vi "ObtainBroadcastEvents.vi"(8 "error in (no error)":errorcluster) -> (0 "error out":errorcluster, 2 "clBroadcastEvents":T1)   [LabVIEW 2017, in "EventModule.lvlib"]
uses:
  EventModule.lvlib
  clBroadcastEvents.ctl
  clEventType.ctl
panel:
  # "These are the default\nBroadcast Events\nfor the cloneable module\n\nIf you want to add your own,create the typedefs in the PublicAPI/Arguments/Broadcast foldr and add event references to the clBroadcastEvents typedef in the Private/Broadcast folder."
  # "If you want to add other Broadcast Events, open this typedef, copy an existing event and rename it to your event name.\n\nNext create a typedef for the  data and put it into PublicAPI/Arguments/Broadcasts"
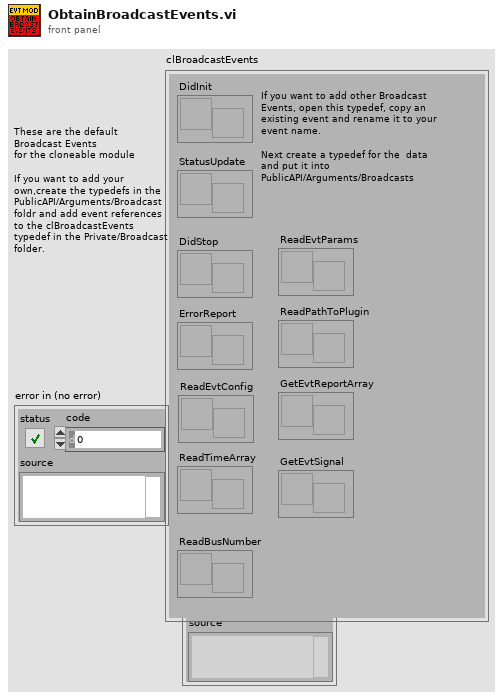
[diagram p1: front panel]
types:
  T1 = typedef "EventModule.lvlib/clBroadcastEvents.ctl" = cluster{"DidInit":refnum<user-event>, "StatusUpdate":refnum<user-event>, "ErrorReport":refnum<user-event>, "DidStop":refnum<user-event>, "ReadEvtConfig":refnum<user-event>, "ReadTimeArray":refnum<user-event>, "ReadEvtParams":refnum<user-event>, "GetEvtReportArray":refnum<user-event>, "ReadPathToPlugin":refnum<user-event>, "GetEvtSignal":refnum<user-event>, "ReadBusNumber":refnum<user-event>}
  T2 = typedef "EventModule.lvlib/clEventType.ctl" = cluster{"ModuleID":i32, "Data":variant}
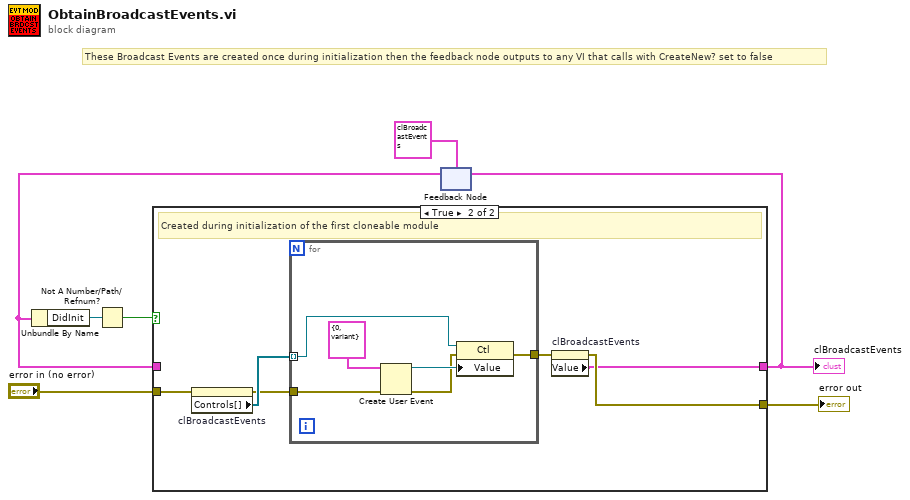
[diagram p0: block diagram]
diagram:
  # "These Broadcast Events are created once during initialization then the feedback node outputs to any VI that calls with CreateNew? set to false"
  n1 = feedback #1(T1 {"DidInit"=refnum, "StatusUpdate"=refnum, "ErrorReport"=refnum, "DidStop"=refnum, "ReadEvtConfig"=refnum, "ReadTimeArray"=refnum, "ReadEvtParams"=refnum, "GetEvtReportArray"=refnum, "ReadPathToPlugin"=refnum, "GetEvtSignal"=refnum, "ReadBusNumber"=refnum} ("Value")) -> (w3:T1)
  n2 = Unbundle By Name(w3) -> ("DidInit"=w2:refnum<user-event>)
  n3 = Not A Number/Path/Refnum?(number/path/refnum=w2) -> (NaN/Path/Refnum?=w1:bool)
  n4 = case shown="True" w1 {
    tunnel: "error in (no error)" -> [w8 w11]
    tunnel: [w8 w15] -> w6
    tunnel: [w9 w14] -> w5
    tunnel: w3 -> [w9 _]
    frame False {
      # "Modules can register to receive these broadcasts or subesquenc cloneable modules can get the events here"
    }
    frame True {
      # "Created during initialization of the first cloneable module"
      n5 = property on="clBroadcastEvents" class="Clust (strict)"(error in=w11) -> (error out=w10:errorcluster, "Controls[]"=w12:refnum<vi>[])  [unwired: 1 in, 1 out]
      n6 = for {
        tunnel: w12 -> [w16] mode=indexing
        tunnel: w10 -> [w21]
        tunnel: [w19] -> w13
        n7 = Create User Event(user event datatype=T2 {"ModuleID"=0, "Data"=variant} ("clBroadcast"), error in=w21) -> (user event=w20:refnum<user-event>, error out=w18:errorcluster)
        n8 = property class="Ctl"(reference=w16, error in=w18, "Value"=w20) -> (error out=w19:errorcluster)  [unwired: 1 out]
      }
      n9 = property on="clBroadcastEvents" class="Clust (strict)"(error in=w13) -> (error out=w15:errorcluster, "Value"=w14:T1)  [unwired: 1 in, 1 out]
    }
  }
  "error out" <- w6
  "clBroadcastEvents" <- w5
  n10 = feedback-in #1(w5) -> ()
